vi "AlphaBetaToDQ_src.vi"(0 "alpha":sgl format="%#_32g", 5 "beta":sgl format="%#_32g", 7 "theta":sgl) -> (4 "direct":sgl, 6 "quadrature":sgl, 13 "sinx":sgl, 14 "cosx":sgl)   [LabVIEW 2017]
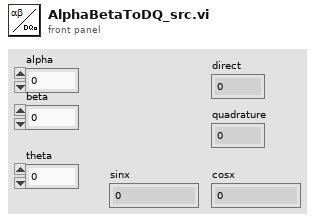
[diagram p1: front panel]
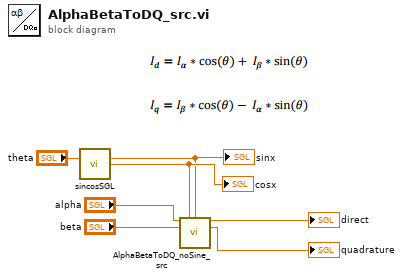
[diagram p0: block diagram]
diagram:
  n1 = call "sincosSGL.vi"("x"="theta") -> ("sinx"=w1:sgl, "cosx"=w2:sgl)  [unwired: 13 in]
  "sinx" <- w1
  "cosx" <- w2
  n2 = call "AlphaBetaToDQ_noSine_src.vi"("alpha"="alpha", "cosx"=w2, "sinx"=w1, "beta"="beta") -> ("direct"=→"direct":sgl, "quadrature"=→"quadrature":sgl)  [unwired: 10 in]
